vi "疫苗信息成簇.vi"(0 "疫苗功能":string="预防virus感染", 4 "是否检验合格":bool=TRUE, 5 "疫苗名":string="anti-virus", 6 "生产负责人":string="DotH", 7 "疫苗编号":i32, 8 "生产地":string="JSCZ", 9 "生产日期":timestamp=timestamp(3639273307.1480513 s since 1904-01-01) format="%<%Y/%m/%d>T", 10 "生产厂家":string="JSFVYY", 11 "是否为第一类疫苗":bool=TRUE) -> (3 "疫苗信息簇":T1 {"生产日期" format="%<%Y/%m/%d>T"})   [LabVIEW 2018]
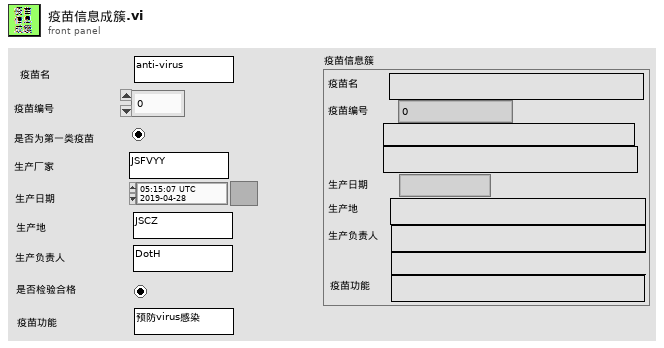
[diagram p1: front panel]
types:
  T1 = typedef "疫苗信息.ctl" = cluster{"疫苗名":string, "疫苗编号":i32, "疫苗类型":string, "生产厂家":string, "生产日期":timestamp, "生产地":string, "生产负责人":string, "是否合格":string, "疫苗功能":string}
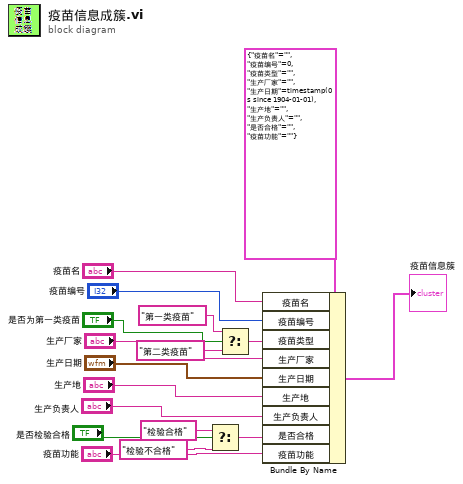
[diagram p0: block diagram]
diagram:
  n1 = Select(t="检验合格", s="是否检验合格", f="检验不合格") -> (s? t:f=w4:string)
  n2 = Select(t="第一类疫苗", s="是否为第一类疫苗", f="第二类疫苗") -> (s? t:f=w8:string)
  n3 = Bundle By Name(cluster=T1 {"疫苗名"="", "疫苗编号"=0, "疫苗类型"="", "生产厂家"="", "生产日期"=timestamp(0 s since 1904-01-01), "生产地"="", "生产负责人"="", "是否合格"="", "疫苗功能"=""} ("疫苗信息"), "疫苗名"="疫苗名", "疫苗编号"="疫苗编号", "疫苗类型"=w8, "生产厂家"="生产厂家", "生产日期"="生产日期", "生产地"="生产地", "生产负责人"="生产负责人", "是否合格"=w4, "疫苗功能"="疫苗功能") -> (→"疫苗信息簇":T1)
